vi "WFS Get Instrument List Info.vi"(8 "error in (no error)":errorcluster {"code" format="%.0x"}, 10 "Instrument List Index":i32 format="%.0g") -> (0 "error out":errorcluster {"code" format="%.0x"}, 1 "In Use":i32, 2 "Device ID":i32, 3 "instrument handle out":refnum<visa-resource-name>, 4 "Instrument Name":string, 5 "Instrument SN":string, 11 "Resource Name":string)   [LabVIEW 2020]
doc: "This VI returns information about one connected WFS instrument selected by Instrument Index."
uses:
  WFS_32.dll
panel:
  in  "instrument handle":refnum<visa-resource-name>
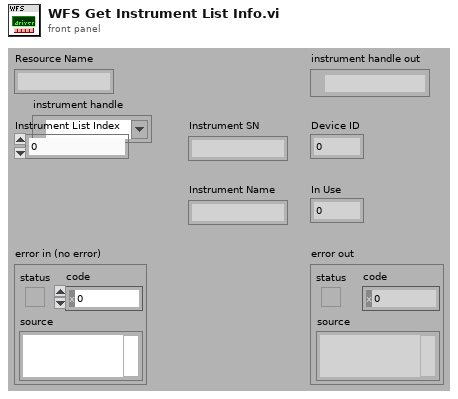
[diagram p1: front panel]
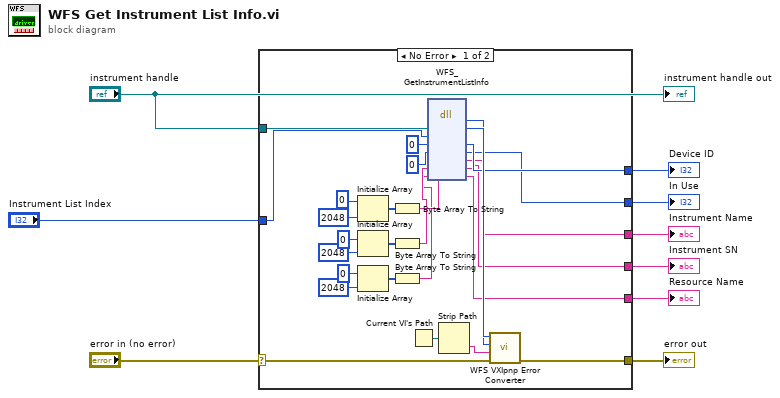
[diagram p0: block diagram]
diagram:
  n1 = case shown="No Error" "error in (no error)" {
    selector: "error in (no error)" -> [w31 w37]
    tunnel: [w30 w37] -> w9
    tunnel: "instrument handle" -> [w35 _]
    tunnel: "Instrument List Index" -> [w29 _]
    tunnel: [w27 _] -> w5
    tunnel: [w25 _] -> w4
    tunnel: [w20 _] -> w3
    tunnel: [w15 _] -> w2
    tunnel: [w10 _] -> w1
    frame No Error {
      n2 = Initialize Array(u8 0 ("element"), 2048 ("dimension size")) -> (w23:u8[])
      n3 = Initialize Array(u8 0 ("element"), 2048 ("dimension size")) -> (w18:u8[])
      n4 = Initialize Array(u8 0 ("element"), 2048 ("dimension size")) -> (w13:u8[])
      n5 = Byte Array To String(unsigned byte array=w23) -> (string=w24:string)
      n6 = Byte Array To String(unsigned byte array=w18) -> (string=w19:string)
      n7 = Byte Array To String(unsigned byte array=w13) -> (string=w14:string)
      n8 = Current VI's Path() -> (path=w36:path)
      n9 = dll-call lib="WFS_*.*" fn="WFS_GetInstrumentListInfo"("Instrument Handle"=w35, "Instrument List Index"=w29, "Device ID"=0, "In Use"=0, "Instrument Name"=w24, "Instrument SN"=w19, "Resource Name"=w14) -> (w33:i32, "Instrument Handle"=w34:u32, "Device ID"=w27:i32, "In Use"=w25:i32, "Instrument Name"=w20:string, "Instrument SN"=w15:string, "Resource Name"=w10:string)  [unwired: 4 in, 2 out]
      n10 = Strip Path(path=w36) -> (name=w32:string)  [unwired: 1 out]
      n11 = call "WFS VXIpnp Error Converter.vi"("error in (no error)"=w31, "Name Of VI (\"\")"=w32, "CVI Error Code (0)"=w33, "instrument handle"=w34) -> ("error out"=w30:errorcluster)  [unwired: 6 in, 1 out]
    }
    frame Error {
    }
  }
  "error out" <- w9
  "Device ID" <- w5
  "In Use" <- w4
  "Instrument Name" <- w3
  "Instrument SN" <- w2
  "Resource Name" <- w1
  "instrument handle out" <- "instrument handle"
